vi "Display_iqa.vi"(9 "connection":refnum<user-event>, 10 "EXIT":refnum<user-event>, 11 "CHANGE":refnum<user-event>) -> ()   [LabVIEW 2017]
uses:
  <vilib>/addons/database/Connection.llb/Conn ObjectReference.ctl
  <vilib>/Utility/miscctls.llb/LVPointTypeDef.ctl
  <vilib>/addons/database/NI_Database_API.lvlib
panel:
  out "TIME:":string
  out "DATE:":string
  out "AFFTER CHECKED":string[][](table)
  out "BEFORE CHECKED":string[][](table)
  # "ELECTRONICS CORPORATION"
  # "BEFORE CHECKED"
  # "AFFTER CHECKED"
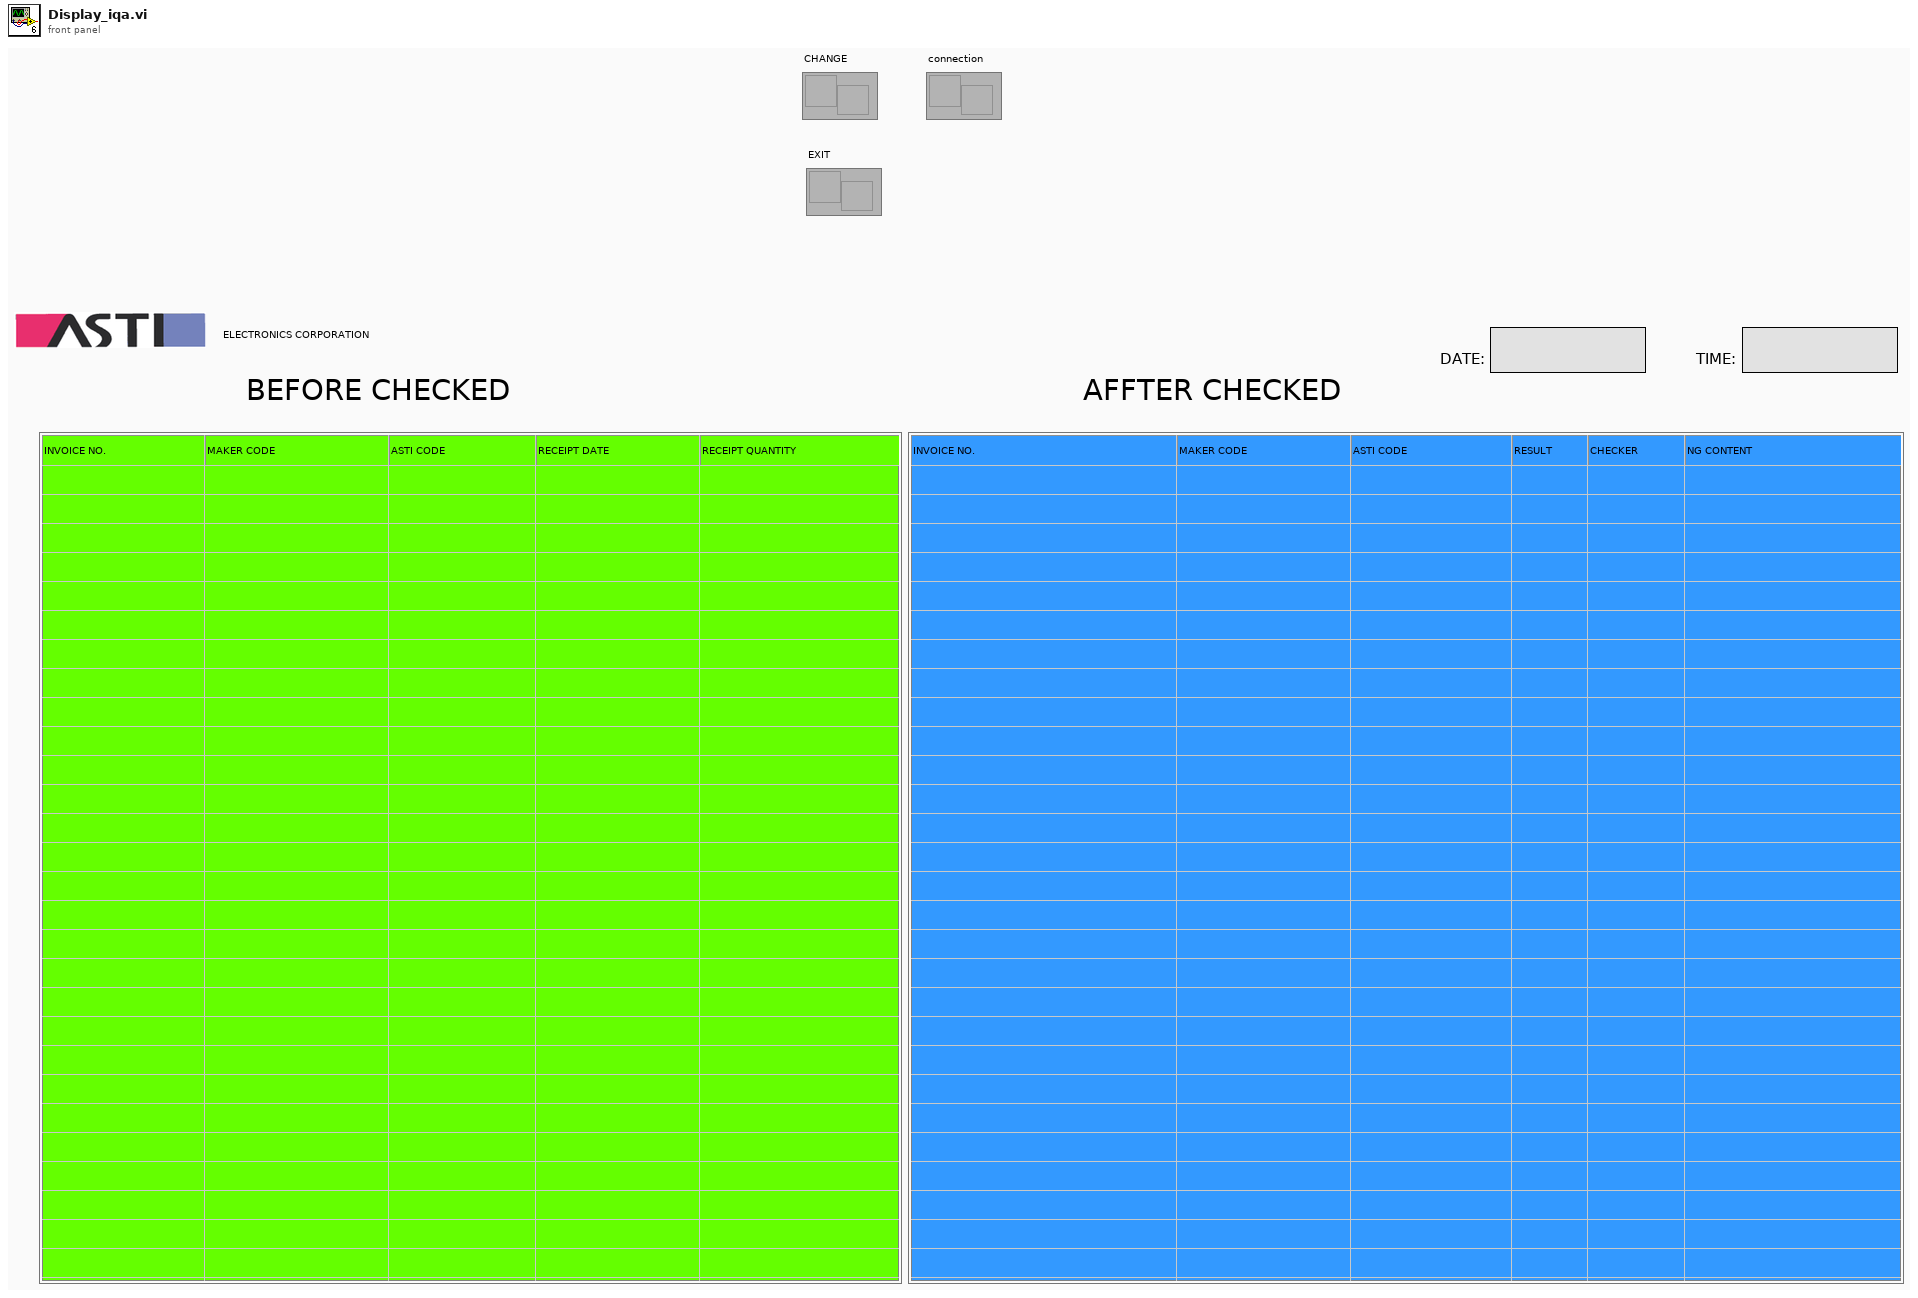
[diagram p1: front panel]
types:
  T1 = typedef "LVPointTypeDef.ctl" = cluster{"Horizontal":i16, "Vertical":i16}
  T2 = typedef "NI_Database_API.lvlib/Conn ObjectReference.ctl" = refnum<k1>
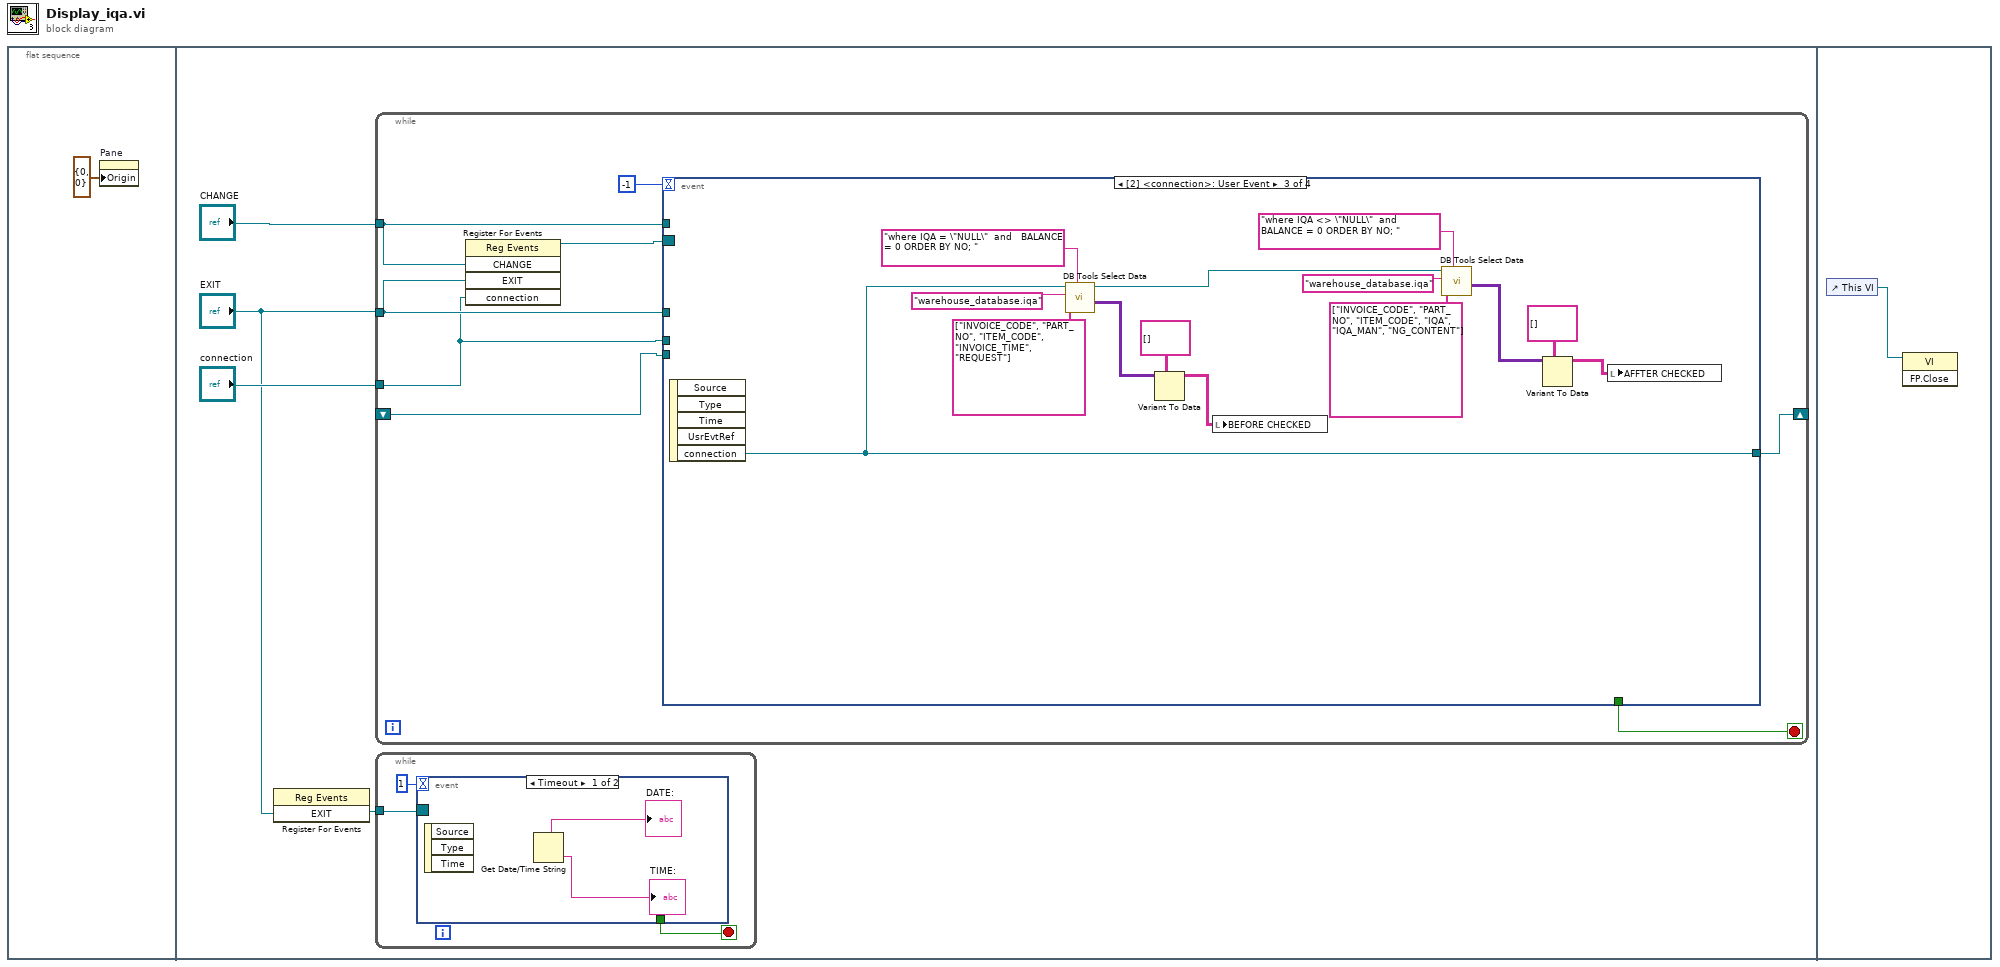
[diagram p0: block diagram]
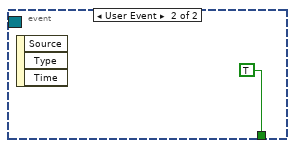
[diagram p2: hidden frame]
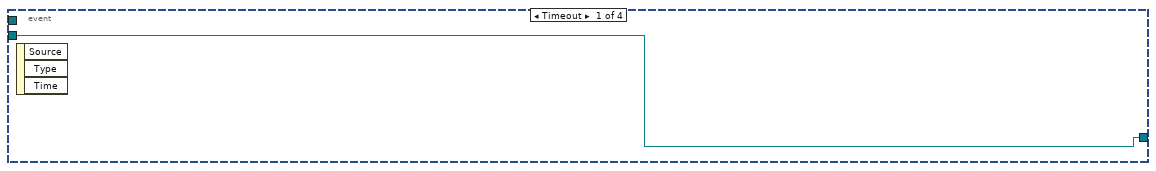
[diagram p3: hidden frame]
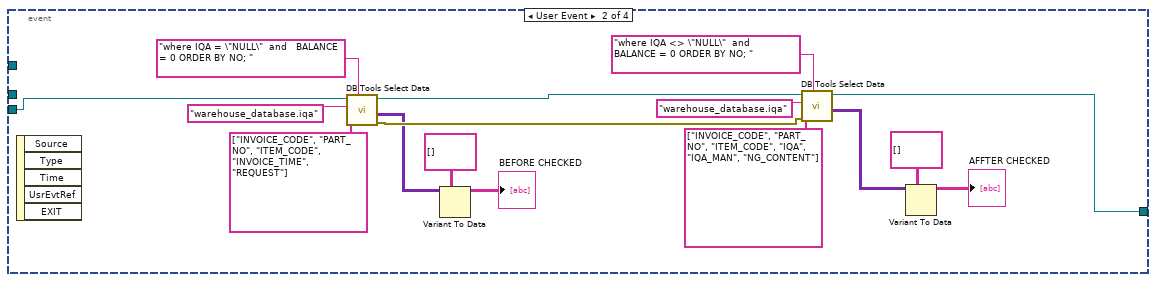
[diagram p4: hidden frame]
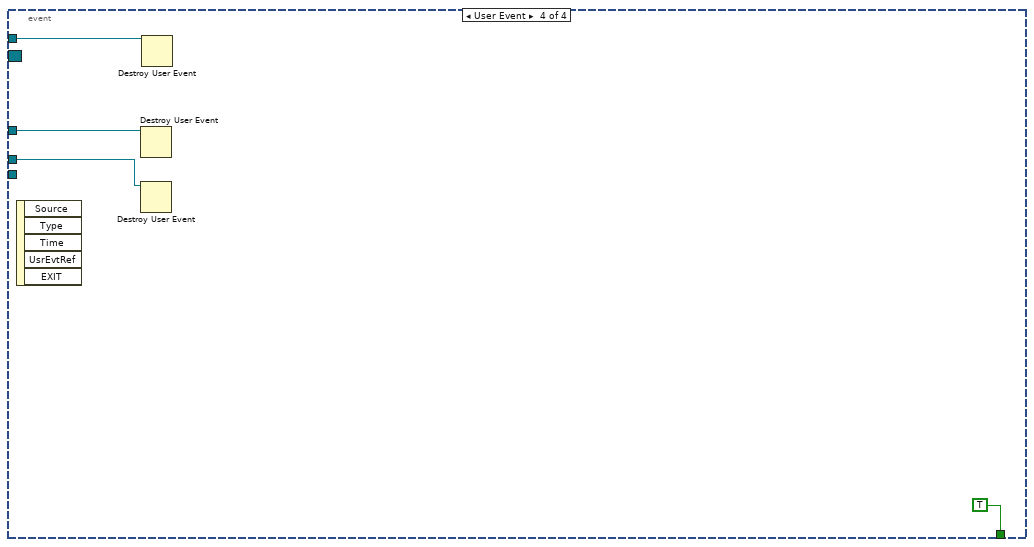
[diagram p5: hidden frame]
diagram:
  n1 = flat-sequence {
    frame #0 {
      n2 = property on="Pane" class="Pane"("Origin"=T1 {"Horizontal"=0, "Vertical"=0}) -> ()  [unwired: 2 in, 2 out]
    }
    frame #1 {
      n3 = register-events("EXIT") -> (reference out=w3:refnum<event-registration>)  [unwired: 2 in, 1 out]
      n4 = while {
        tunnel: "EXIT" -> [w16]
        tunnel: "CHANGE" -> [w15]
        shift-right: [w14] -> _
        shift-left: _ -> [w13]
        tunnel: "connection" -> [w12]
        stop <- w17 stop-if-true
        n5 = register-events(w15, w16, w12) -> (reference out=w19:refnum<event-registration>)  [unwired: 2 in, 1 out]
        n6 = event shown="[2] <connection>: User Event" {
          selector: w19 -> [_ _ _ _]
          dyn-events: _ -> [_ _ _ _]
          timeout: -1 -> [_ _ _ _]
          tunnel: w13 -> [w20 w36 _ _]
          tunnel: [_ _ _ TRUE] -> w17
          tunnel: w15 -> [_ _ _ w53]
          tunnel: w16 -> [_ _ _ w52]
          tunnel: [w20 w21 w40 _] -> w14
          tunnel: w12 -> [_ _ _ w51]
          event Timeout {
            n7 = event-data() -> ()  [unwired: 1 in, 3 out]
          }
          event User Event {
            n8 = event-data() -> ()  [unwired: 1 in, 5 out]
            n9 = call <vilib>:"DB Tools Select Data.vi"("condition"="where IQA = \"NULL\"  and   BALANCE = 0 ORDER BY NO; ", "columns"=string[] ["INVOICE_CODE", "PART_NO", "ITEM_CODE", "INVOICE_TIME", "REQUEST"], "table"="warehouse_database.iqa", "connection reference"=w36) -> ("error out"=w28:errorcluster, "data"=w27:variant[][], "connection reference out"=w29:T2)  [unwired: 2 in]
            n10 = Variant To Data(type=string[][] [], Variant=w27) -> (data=→"BEFORE CHECKED":string[][])  [unwired: 1 in, 1 out]
            n11 = call <vilib>:"DB Tools Select Data.vi"("condition"="where IQA <> \"NULL\"  and   BALANCE = 0 ORDER BY NO; ", "error in (no error)"=w28, "columns"=string[] ["INVOICE_CODE", "PART_NO", "ITEM_CODE", "IQA", "IQA_MAN", "NG_CONTENT"], "table"="warehouse_database.iqa", "connection reference"=w29) -> ("data"=w23:variant[][], "connection reference out"=w21:T2)  [unwired: 1 in, 1 out]
            n12 = Variant To Data(type=string[][] [], Variant=w23) -> (data=→"AFFTER CHECKED":string[][])  [unwired: 1 in, 1 out]
          }
          event User Event {
            n13 = event-data() -> ("connection"=w40:T2)  [unwired: 1 in, 4 out]
            n14 = call <vilib>:"DB Tools Select Data.vi"("condition"="where IQA = \"NULL\"  and   BALANCE = 0 ORDER BY NO; ", "columns"=string[] ["INVOICE_CODE", "PART_NO", "ITEM_CODE", "INVOICE_TIME", "REQUEST"], "table"="warehouse_database.iqa", "connection reference"=w40) -> ("data"=w47:variant[][], "connection reference out"=w39:T2)  [unwired: 2 in, 1 out]
            n15 = Variant To Data(type=string[][] [], Variant=w47) -> (data=w38:string[][])  [unwired: 1 in, 1 out]
            n16 = local write "BEFORE CHECKED"(w38) -> ()
            n17 = call <vilib>:"DB Tools Select Data.vi"("condition"="where IQA <> \"NULL\"  and   BALANCE = 0 ORDER BY NO; ", "columns"=string[] ["INVOICE_CODE", "PART_NO", "ITEM_CODE", "IQA", "IQA_MAN", "NG_CONTENT"], "table"="warehouse_database.iqa", "connection reference"=w39) -> ("data"=w41:variant[][])  [unwired: 2 in, 2 out]
            n18 = Variant To Data(type=string[][] [], Variant=w41) -> (data=w37:string[][])  [unwired: 1 in, 1 out]
            n19 = local write "AFFTER CHECKED"(w37) -> ()
          }
          event User Event {
            n20 = event-data() -> ()  [unwired: 1 in, 5 out]
            n21 = Destroy User Event(user event=w52) -> ()  [unwired: 1 in, 1 out]
            n22 = Destroy User Event(user event=w51) -> ()  [unwired: 1 in, 1 out]
            n23 = Destroy User Event(user event=w53) -> ()  [unwired: 1 in, 1 out]
          }
        }
      }
      n24 = while {
        tunnel: w3 -> [w8]
        stop <- w7 stop-if-true
        n25 = event shown="[0] Timeout" {
          selector: w8 -> [_ _]
          dyn-events: _ -> [_ _]
          timeout: 1 -> [_ _]
          tunnel: [_ TRUE] -> w7
          event Timeout {
            n26 = event-data() -> ()  [unwired: 1 in, 3 out]
            n27 = Get Date/Time String() -> (date string=→"DATE:":string, time string=→"TIME:":string)  [unwired: 3 in]
          }
          event User Event {
            n28 = event-data() -> ()  [unwired: 1 in, 3 out]
          }
        }
      }
    }
    frame #2 {
      n29 = control-ref of="This VI"() -> (w55:refnum<vi>)
      n30 = invoke class="VI" method="FP.Close"(reference=w55) -> ()  [unwired: 2 in, 3 out]
    }
  }
